vi "Trig OP Setup-Parser.vi"(0 "Triggers output setup to save":T1=[{"Name"="", "Output?"=FALSE, "Output terminal"="/PXI1Slot6/PFI0", "PXI backplane line"="/PXI1Slot6/PXI_Trig0", "Pulse width (us)"=20}, {"Name"="", "Output?"=FALSE, "Output terminal"="/PXI1Slot6/PFI0", "PXI backplane line"="/PXI1Slot6/PXI_Trig0", "Pulse width (us)"=20}, {"Name"="", "Output?"=FALSE, "Output terminal"="/PXI1Slot6/PFI0", "PXI backplane line"="/PXI1Slot6/PXI_Trig0", "Pulse width (us)"=20}, {"Name"="", "Output?"=FALSE, "Output terminal"="/PXI1Slot6/PFI0", "PXI backplane line"="/PXI1Slot6/PXI_Trig0", "Pulse width (us)"=20}, {"Name"="", "Output?"=FALSE, "Output terminal"="/PXI1Slot6/PFI0", "PXI backplane line"="/PXI1Slot6/PXI_Trig0", "Pulse width (us)"=20}, {"Name"="", "Output?"=FALSE, "Output terminal"="/PXI1Slot6/PFI0", "PXI backplane line"="/PXI1Slot6/PXI_Trig0", "Pulse width (us)"=20}] {"Pulse width (us)" min=10 max=5000 step=1 format="%.0fµs"}) -> (16 "Keys setup":T3=[{"key"="Control FPGA.MAC address", "Save?"=TRUE, "Default"="AABBCCDDEEFF"}, {"key"="DAQ FPGA.Target", "Save?"=TRUE, "Default"="RIO0"}, {"key"="XY Stage.COM port", "Save?"=TRUE, "Default"="COM7"}, {"key"="DAQmx Chan.Pockels Control", "Save?"=TRUE, "Default"=""}, {"key"="DAQmx Chan.Hard Shutter", "Save?"=TRUE, "Default"=""}, {"key"="DAQmx Chan.PMT 1", "Save?"=TRUE, "Default"=""}, {"key"="DAQmx Chan.PMT 2", "Save?"=TRUE, "Default"=""}, {"key"="DAQmx Chan.Encoder Trigger", "Save?"=TRUE, "Default"=""}, {"key"="DAQmx Chan.Optional Trigger 1", "Save?"=TRUE, "Default"=""}, {"key"="DAQmx Chan.Optional Trigger 2", "Save?"=TRUE, "Default"=""}, {"key"="DAQmx Chan.Optional Trigger 3", "Save?"=TRUE, "Default"=""}], 17 "Values.Strings":string[](array[string]))   [LabVIEW 2013]
uses:
  Typedefs/Ini file interface (String).ctl
  Peripherals Control/Triggers/Typedefs/Triggers output setup.ctl
  Peripherals Control/Triggers/Typedefs/Trigger setup element cluster.ctl
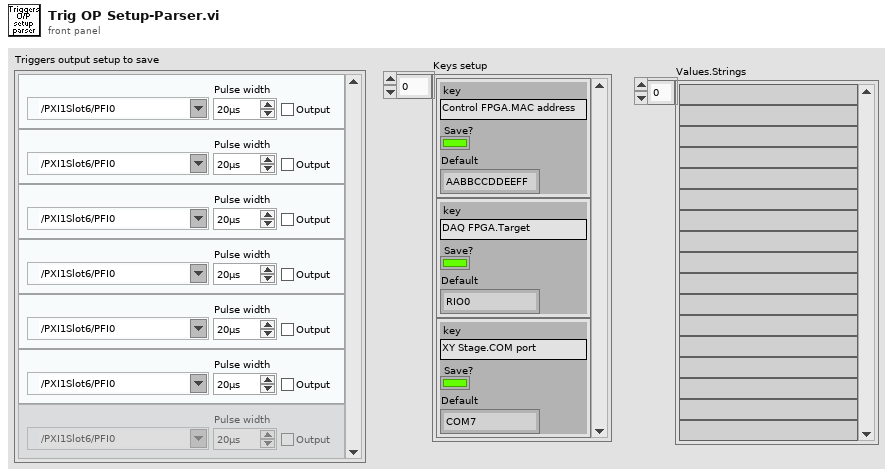
[diagram p1: front panel]
types:
  T1 = typedef "Triggers output setup.ctl" = T2[]
  T2 = typedef "Trigger setup element cluster.ctl" = cluster{"Name":string, "Output?":bool, "Output terminal":tag, "PXI backplane line":tag, "Pulse width (us)":u16}
  T3 = typedef "Ini file interface (String).ctl" = cluster{"key":string, "Save?":bool, "Default":string}[]
  T4 = cluster{"key":string, "Save?":bool, "Default":string}[]
  T5 = cluster{"Name":string, "Output":bool, "Output terminal":tag, "PXI backplane line":tag, "Pulse width":u16}[]
  T6 = cluster{"key":string, "Save?":bool, "Default":string}
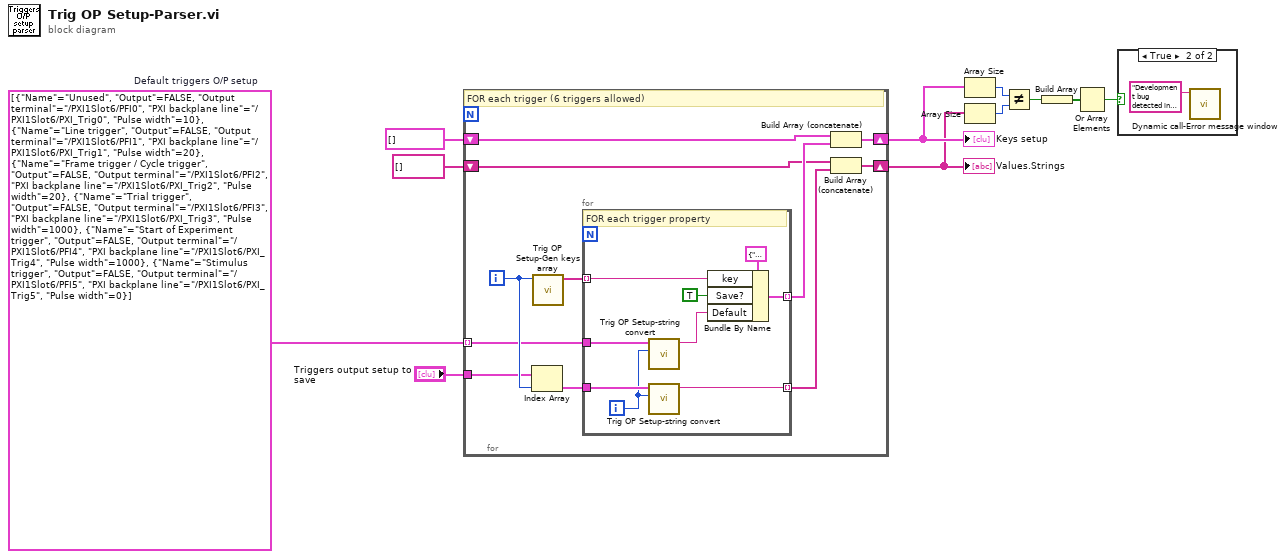
[diagram p0: block diagram]
diagram:
  w1 = T5 [{"Name"="Unused", "Output"=FALSE, "Output terminal"="/PXI1Slot6/PFI0", "PXI backplane line"="/PXI1Slot6/PXI_Trig0", "Pulse width"=10}, {"Name"="Line trigger", "Output"=FALSE, "Output terminal"="/PXI1Slot6/PFI1", "PXI backplane line"="/PXI1Slot6/PXI_Trig1", "Pulse width"=20}, {"Name"="Frame trigger / Cycle trigger", "Output"=FALSE, "Output terminal"="/PXI1Slot6/PFI2", "PXI backplane line"="/PXI1Slot6/PXI_Trig2", "Pulse width"=20}, {"Name"="Trial trigger", "Output"=FALSE, "Output terminal"="/PXI1Slot6/PFI3", "PXI backplane line"="/PXI1Slot6/PXI_Trig3", "Pulse width"=1000}, {"Name"="Start of Experiment trigger", "Output"=FALSE, "Output terminal"="/PXI1Slot6/PFI4", "PXI backplane line"="/PXI1Slot6/PXI_Trig4", "Pulse width"=1000}, {"Name"="Stimulus trigger", "Output"=FALSE, "Output terminal"="/PXI1Slot6/PFI5", "PXI backplane line"="/PXI1Slot6/PXI_Trig5", "Pulse width"=0}]  # Default triggers O/P setup
  n1 = for {
    tunnel: "Triggers output setup to save" -> [w13]
    shift-right: [w19] -> w3
    shift-left: T4 [] -> [w18]
    shift-right: [w16] -> w2
    shift-left: string[] [] -> [w15]
    tunnel: w1 -> [w14] mode=indexing
    i -> [w21]
    # "FOR each trigger (6 triggers allowed)"
    n2 = Index Array(array=w13, index=w21) -> (element=w12:T2)
    n3 = call "Trig OP Setup-Gen keys array.vi"("Trigger index (FOR loop index)"=w21) -> ("Keys array for each trigger"=w22:string[])  [unwired: 10 in]
    n4 = for {
      tunnel: w22 -> [w31] mode=indexing
      tunnel: w14 -> [w30]
      tunnel: [w26] -> w20 mode=indexing
      tunnel: w12 -> [w25]
      tunnel: [w24] -> w17 mode=indexing
      i -> [w23]
      # "FOR each trigger property"
      n5 = call "Trig OP Setup-string convert.vi"("FOR loop index"=w23, "Trigger setup element"=w30) -> ("String"=w27:string)  [unwired: 9 in]
      n6 = call "Trig OP Setup-string convert.vi"("FOR loop index"=w23, "Trigger setup element"=w25) -> ("String"=w24:string)  [unwired: 9 in]
      n7 = Bundle By Name(cluster=T6 {"key"="", "Save?"=TRUE, "Default"=""}, "key"=w31, "Save?"=TRUE, "Default"=w27) -> (w26:T6)
    }
    n8 = Build Array (concatenate)(w18, w20) -> (w19:T4)
    n9 = Build Array (concatenate)(w15, w17) -> (w16:string[])
  }
  "Keys setup" <- w3
  "Values.Strings" <- w2
  n10 = Array Size(array=w3) -> (size(s)=w8:i32)
  n11 = Array Size(array=w2) -> (size(s)=w7:i32)
  n12 = Not Equal?(x=w8, y=w7) -> (x != y?=w4:bool)
  n13 = Build Array(w4) -> (w6:bool[])
  n14 = Or Array Elements(Boolean array=w6) -> (logical OR=w5:bool)
  n15 = case shown="True" w5 {
    frame False {
    }
    frame True {
      n16 = call "Dynamic call-Error message window.vi"("Error Message"="Development bug detected in the \"Trig OP Setup-Parser.vi\".\nPlease correct the set up in this VI.") -> ()  [unwired: 10 in, 1 out]
    }
  }
